vi "subPanel - Write Value.vi"(6 "Val(Sgnl)":bool, 8 "Error In":errorcluster, 10 "CtlRef Controls[]":refnum<vi>[](array[refnum]), 11 "Pnl Control":refnum<vi>) -> (0 "Error Out":errorcluster, 2 "CtlRef Controls[]":refnum<vi>[](array[refnum]), 3 "Pnl Control":refnum<vi>)   [LabVIEW 2013]
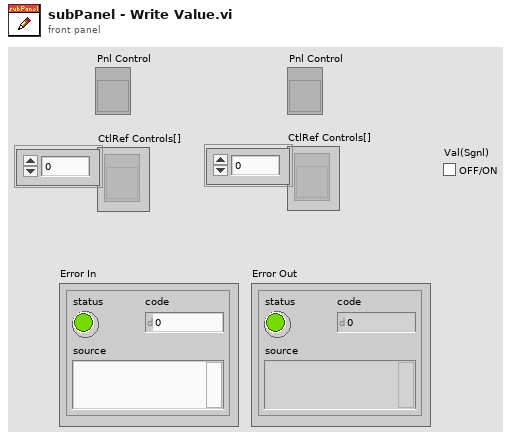
[diagram p1: front panel]
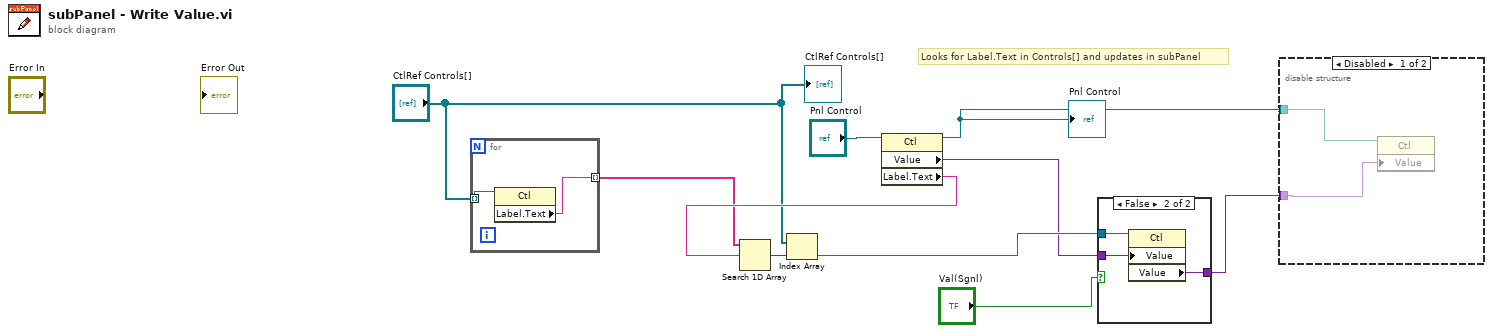
[diagram p0: block diagram]
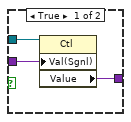
[diagram p2: hidden frame]
diagram:
  # "Looks for Label.Text in Controls[] and updates in subPanel"
  n1 = for {
    tunnel: "CtlRef Controls[]" -> [w12] mode=indexing
    tunnel: [w11] -> w2 mode=indexing
    n2 = property class="Ctl"(reference=w12) -> ("Label.Text"=w11:string)  [unwired: 1 in, 2 out]
  }
  n3 = property class="Ctl"(reference="Pnl Control") -> (reference out=w6:refnum<vi>, "Value"=w7:variant, "Label.Text"=w4:string)  [unwired: 1 in, 1 out]
  "Pnl Control" <- w6
  n4 = Search 1D Array(1D array=w2, element=w4) -> (index of element=w9:i32)  [unwired: 1 in]
  n5 = Index Array(array="CtlRef Controls[]", index=w9) -> (element=w10:refnum<vi>)
  n6 = case shown="False" "Val(Sgnl)" {
    tunnel: w10 -> [w15 w18]
    tunnel: w7 -> [w14 w17]
    tunnel: [w13 w16] -> w5
    frame True {
      n7 = property class="Ctl"(reference=w15, "Val(Sgnl)"=w14) -> ("Value"=w13:variant)  [unwired: 1 in, 2 out]
    }
    frame False {
      n8 = property class="Ctl"(reference=w18, "Value"=w17) -> ("Value"=w16:variant)  [unwired: 1 in, 2 out]
    }
  }
  n9 = disable-structure shown="Disabled" {
    disable-tunnel: w6 -> [w20 _]
    disable-tunnel: w5 -> [w19 _]
    frame Disabled {
      n10 = property class="Ctl"(reference=w20, "Value"=w19) -> ()  [unwired: 1 in, 2 out]
    }
    frame Enabled {
    }
  }
  "CtlRef Controls[]" <- "CtlRef Controls[]"
